vi "Microwave Oven.vi"(0 "Key_Pad":T2 caption="Key Pad", 5 "Stop":bool, 7 "Door_Open":bool caption="Door Open") -> (4 "Display_Panel":string caption="Display Panel", 6 "Recipe":string[][](table), 8 "Oven_Data_Display":T1 caption="Microwave Oven")   [LabVIEW 2023]
doc: "This VI is the Main VI that performs the oven operations."
uses:
  Controls/Key_Pad.ctl
  Controls/Oven_Data_Display.ctl
  Controls/Oven_Data.ctl
  Controls/Timer_Operation_Select.ctl
  Controls/Timer_Data.ctl
  Controls/Queue_Operation_Select.ctl
  <vilib>/Utility/file.llb/Read Delimited Spreadsheet (string).vi
panel:
  out "Error_Out":errorcluster
  in  "Error_In":errorcluster
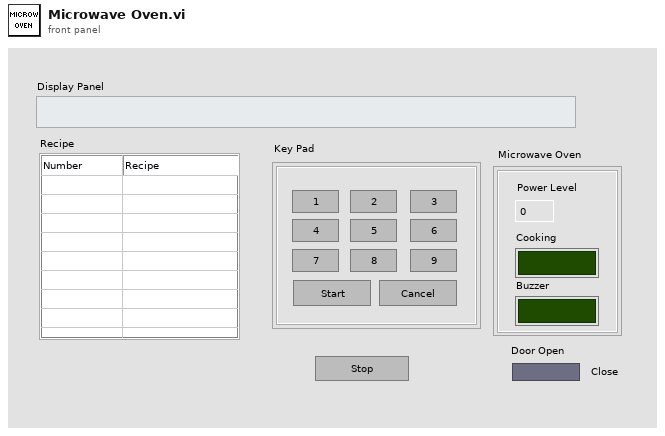
[diagram p1: front panel]
types:
  T1 = typedef "Oven_Data_Display.ctl" = cluster{"Power_Level":i32, "Cooking":bool, "Buzzer":bool}
  T2 = typedef "Key_Pad.ctl" = cluster{"One":bool, "Two":bool, "Three":bool, "Four":bool, "Five":bool, "Six":bool, "Seven":bool, "Eight":bool, "Nine":bool, "Start":bool, "Cancel":bool}
  T3 = typedef "Queue_Operation_Select.ctl" = enum16{"Obtain_Queue", "Enqueue", "Enqueue_at_First", "Enqueue_N", "Dequeue", "Flush_Queue", "Release_Queue"}
  T4 = typedef "Oven_Data.ctl" = cluster{"Recipe_Data":string[][], "Display_Message":string, "Recipe_Code":i32, "Start?":bool, "Cancel?":bool, "TimeOut?":bool, "Door_Open?":bool, "Cooking_Completed?":bool, "Current_Stage":i32, "Timer_Operation_Select":T5, "Oven_Data_Display":T1, "Recipe_Data_Dispaly":string[][], "Total_Stage":i32, "Timer_Data":T6, "Recipe_Selected":string}
  T5 = typedef "Timer_Operation_Select.ctl" = enum16{"Start_Timer", "Pause_Timer", "Stop_Timer", "CheckOut_Timer"}
  T6 = typedef "Timer_Data.ctl" = cluster{"Present_Time":dbl, "Start?":bool, "Time_Before_Pause":dbl, "Time_Required":dbl, "Time":dbl}
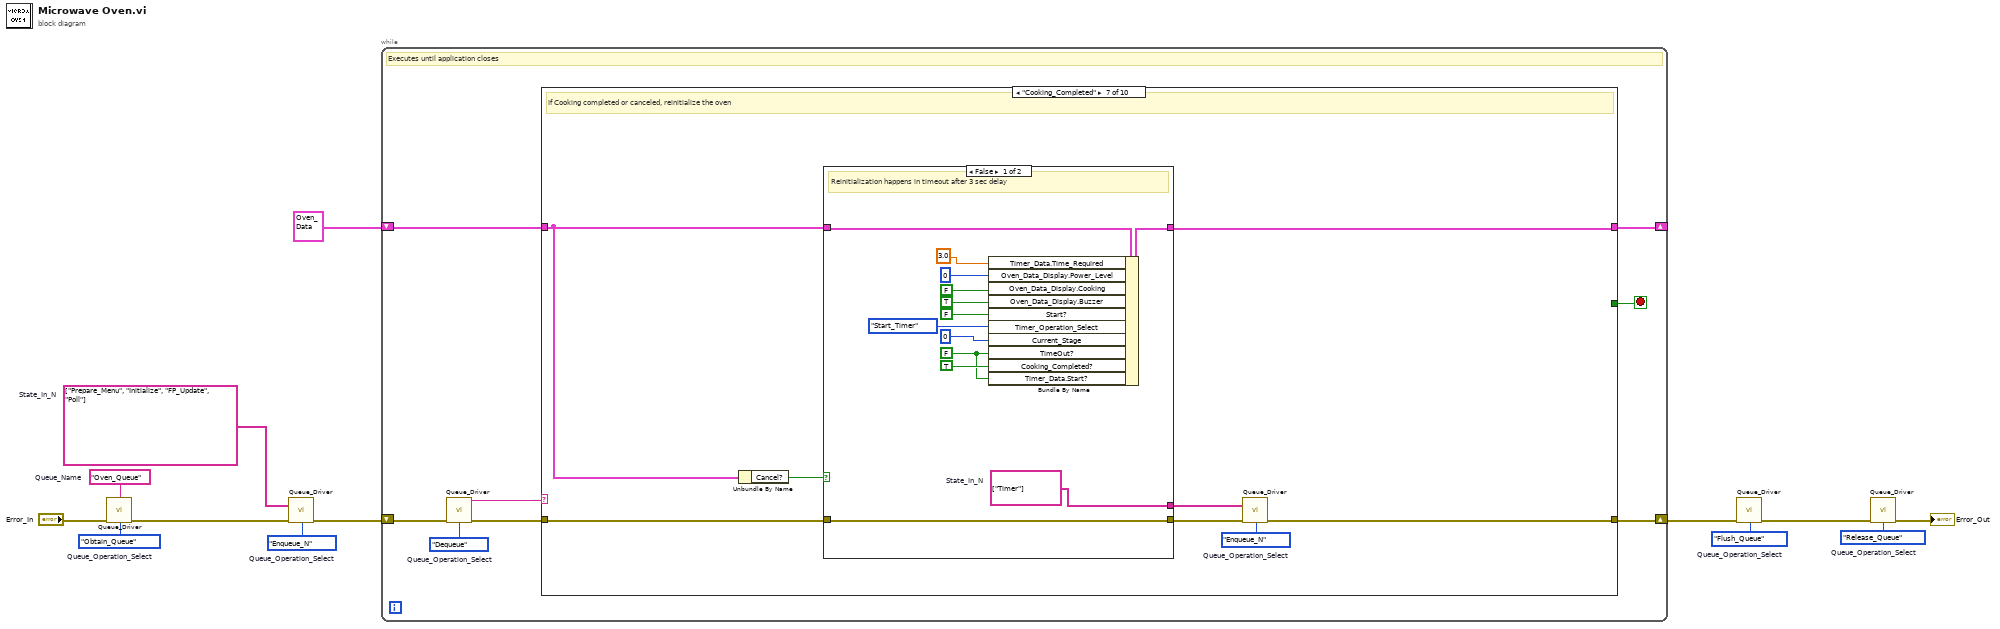
[diagram p0: block diagram]
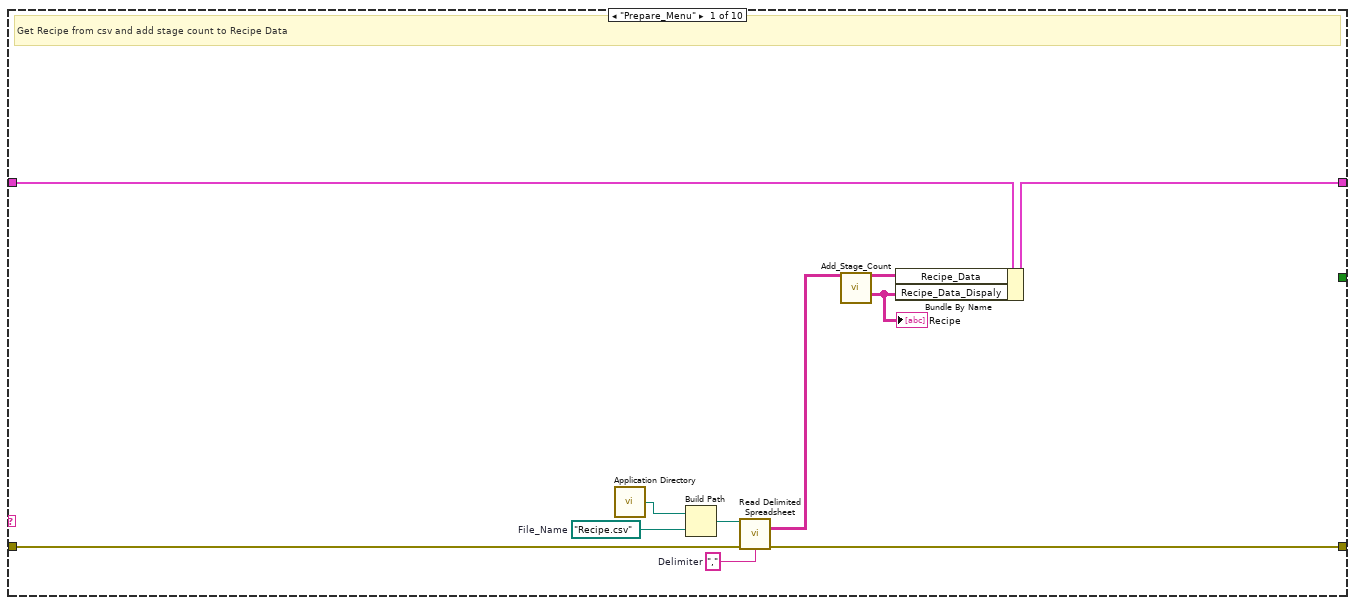
[diagram p2: hidden frame]
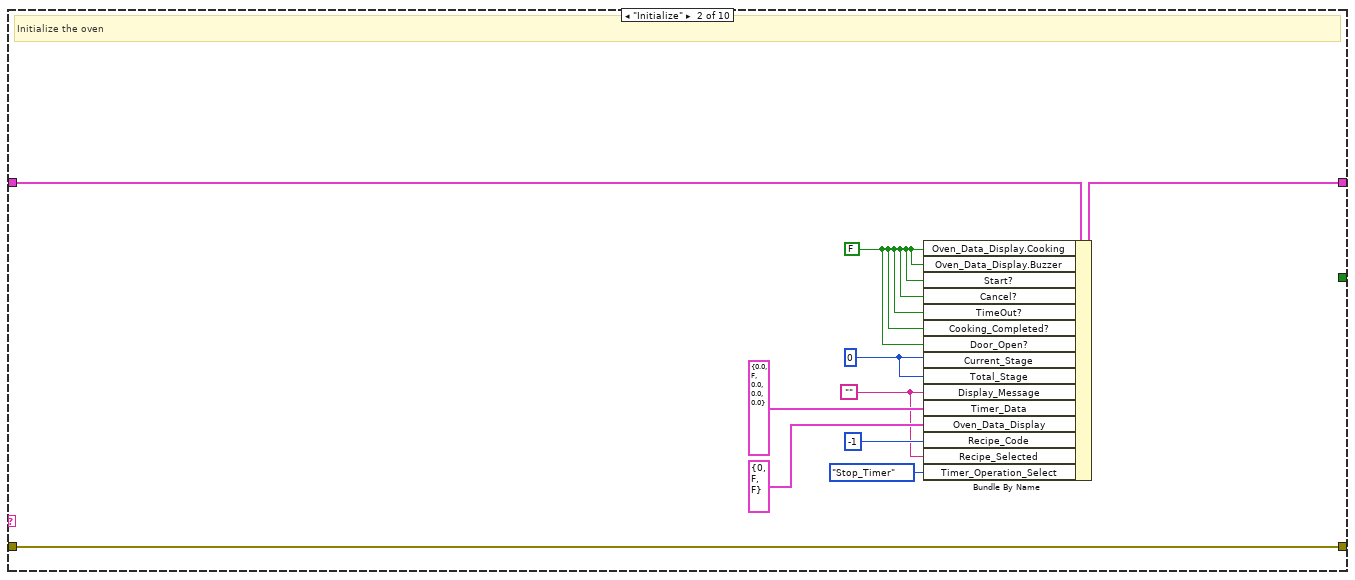
[diagram p3: hidden frame]
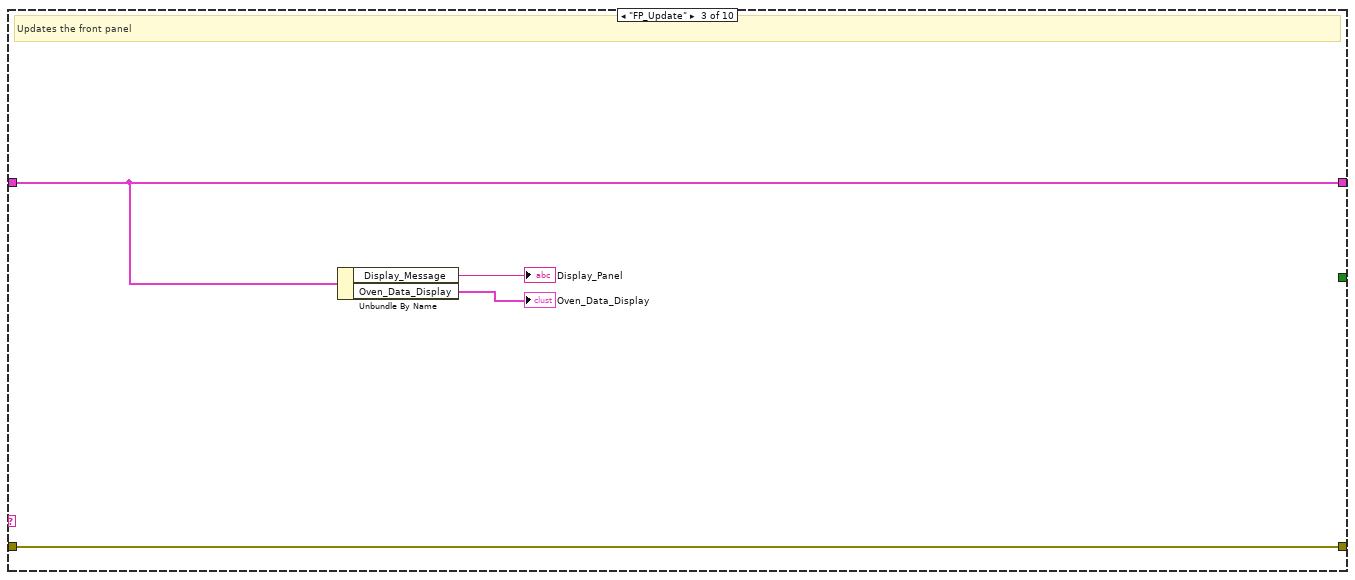
[diagram p4: hidden frame]
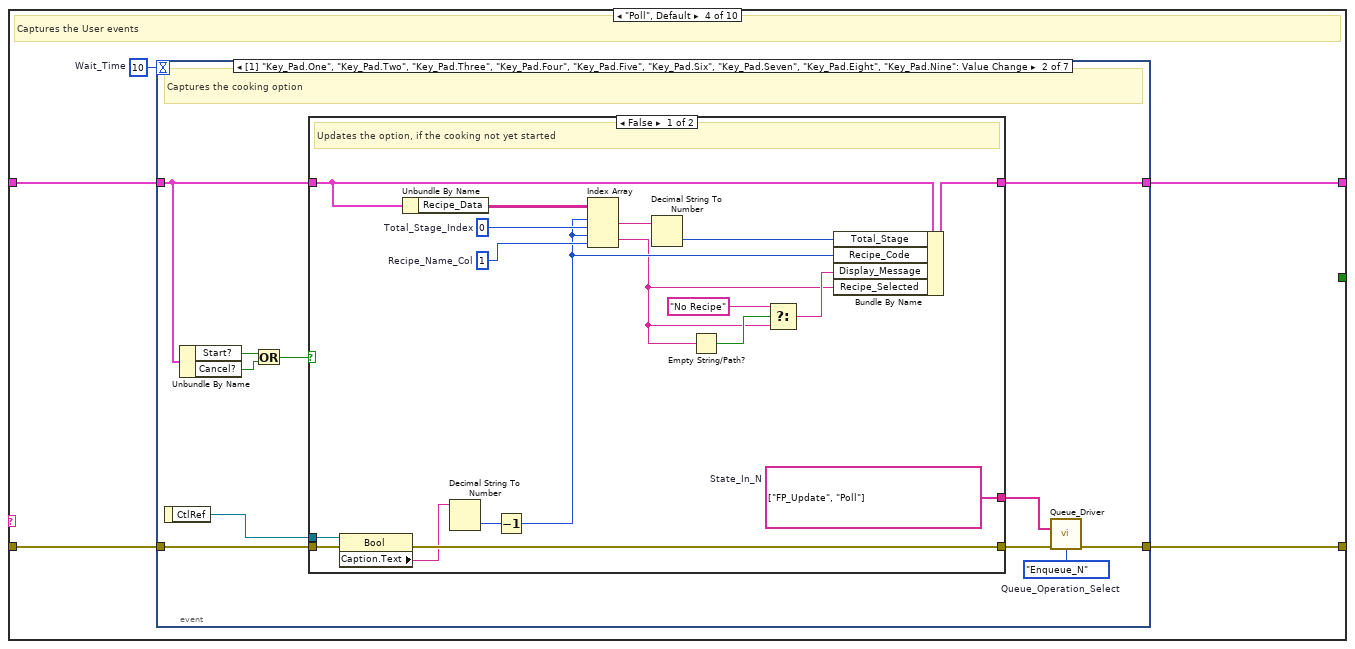
[diagram p5: hidden frame]
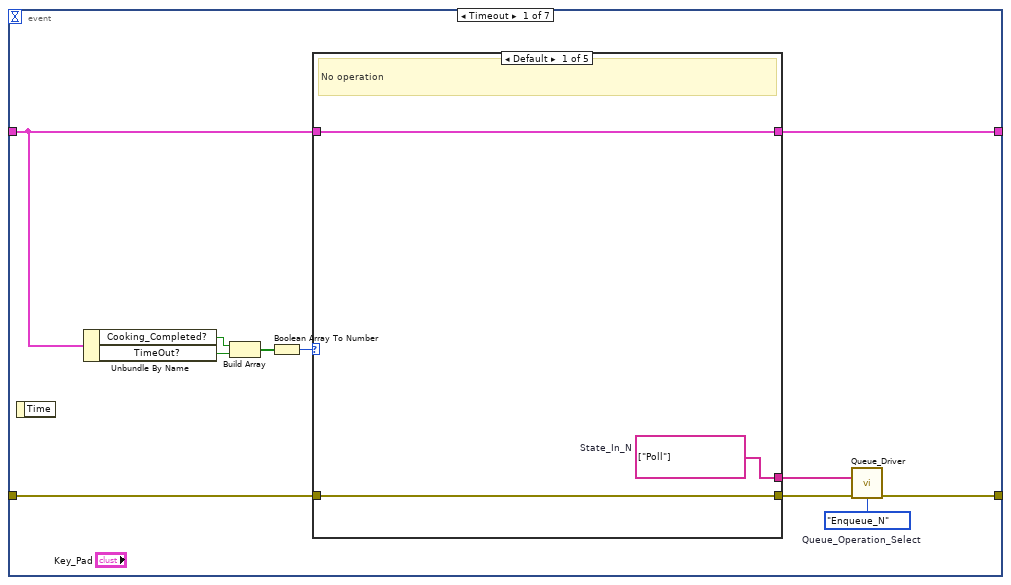
[diagram p6: hidden frame]
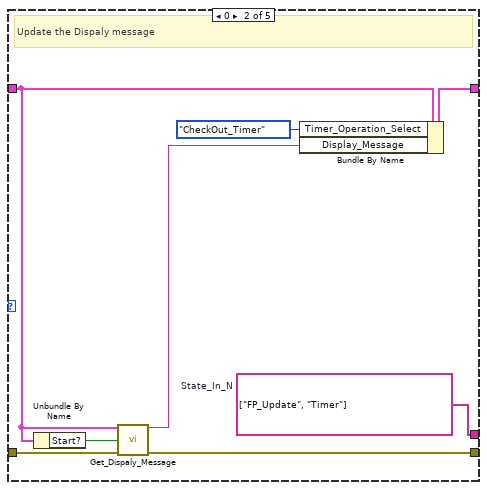
[diagram p7: hidden frame]
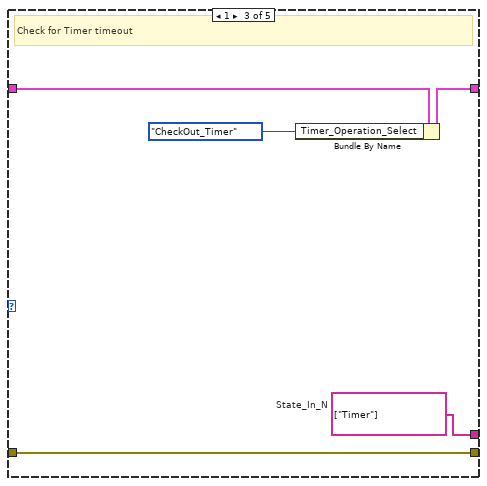
[diagram p8: hidden frame]
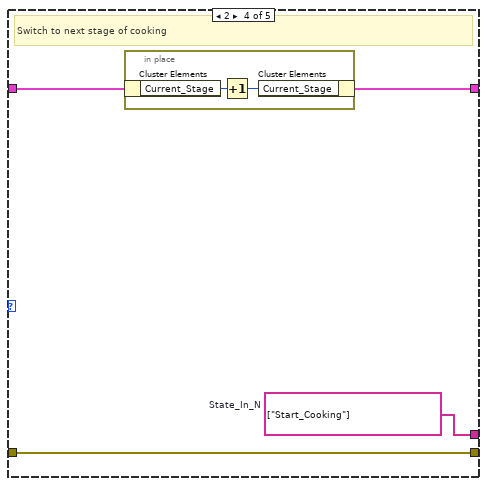
[diagram p9: hidden frame]
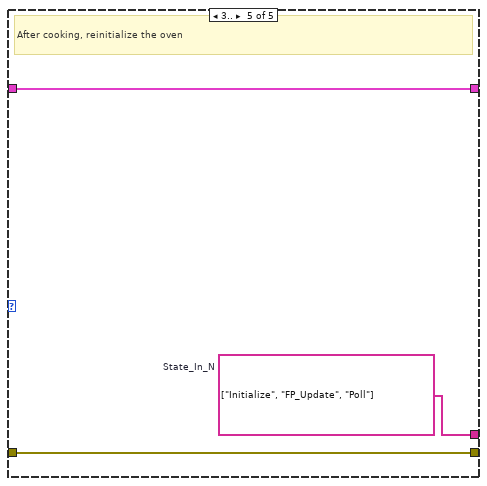
[diagram p10: hidden frame]
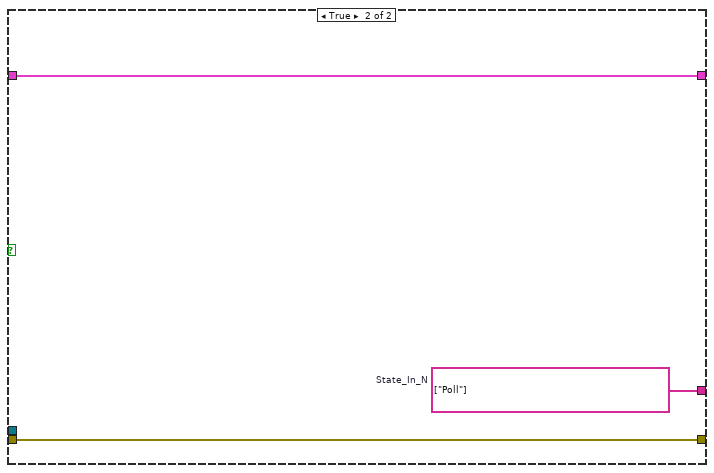
[diagram p11: hidden frame]
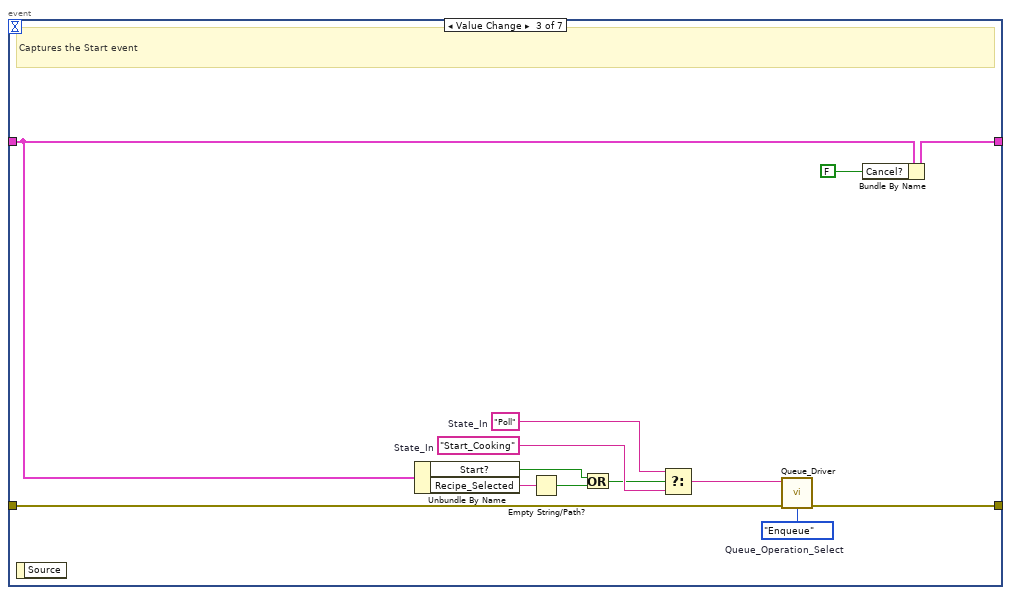
[diagram p12: hidden frame]
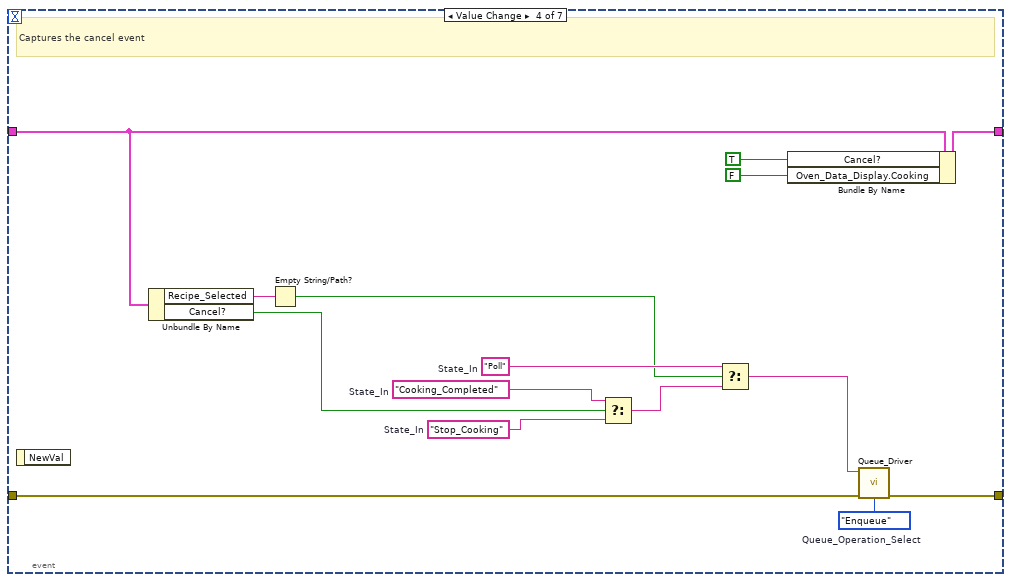
[diagram p13: hidden frame]
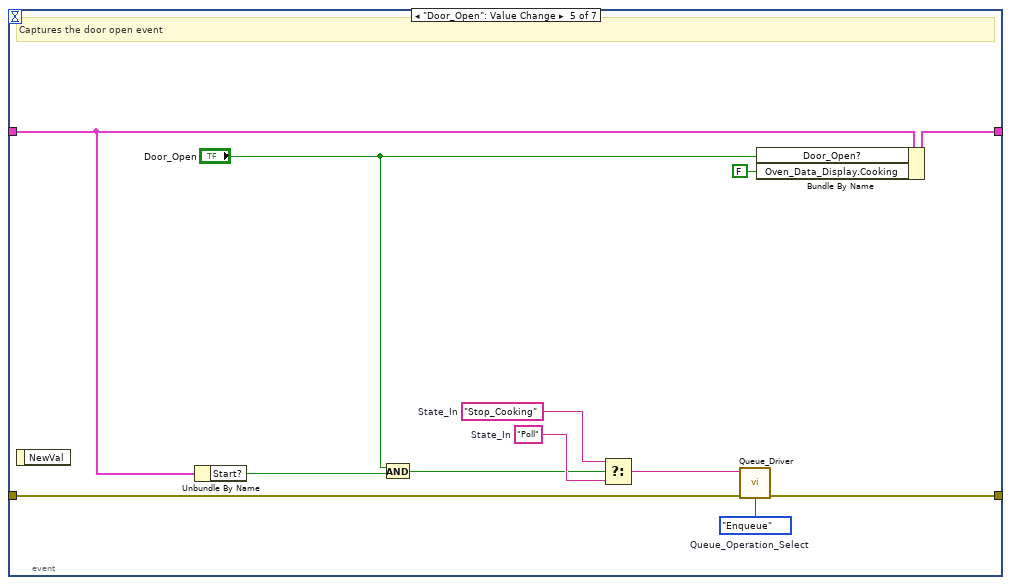
[diagram p14: hidden frame]
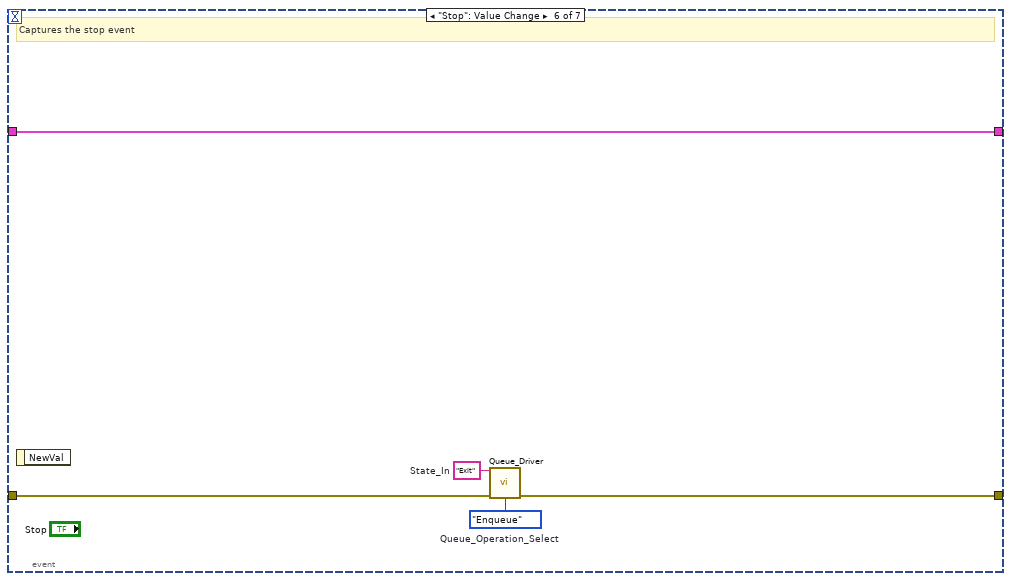
[diagram p15: hidden frame]
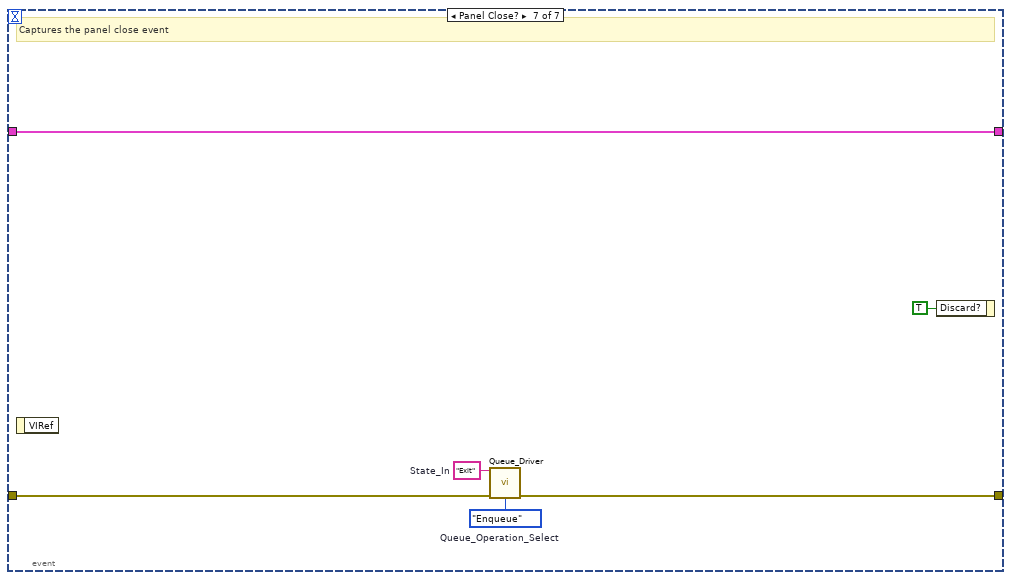
[diagram p16: hidden frame]
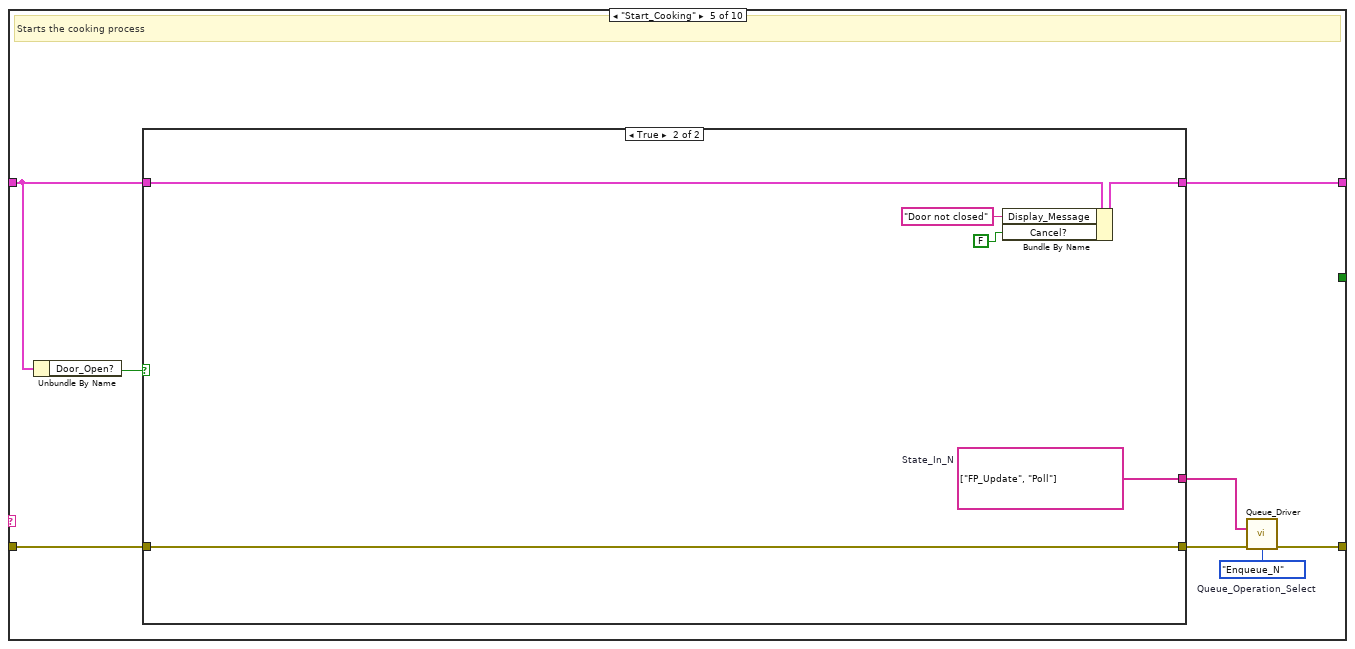
[diagram p17: hidden frame]
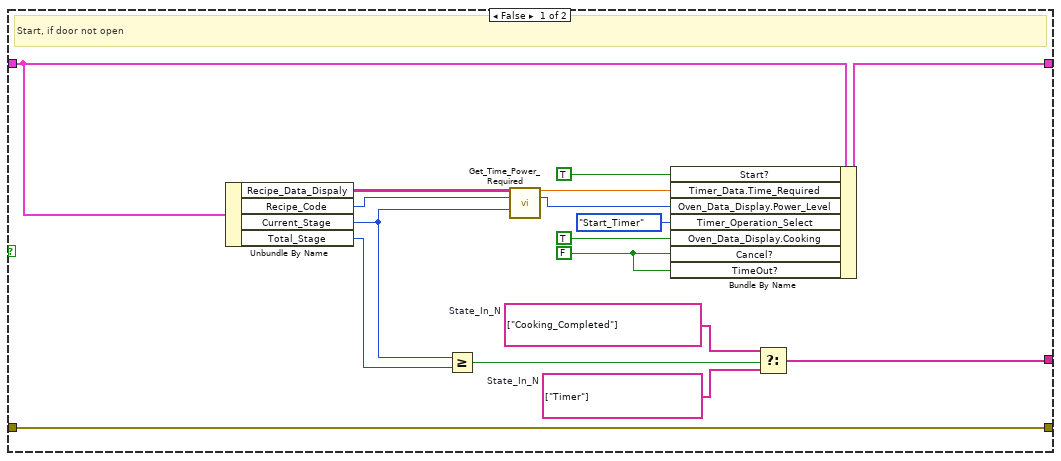
[diagram p18: hidden frame]
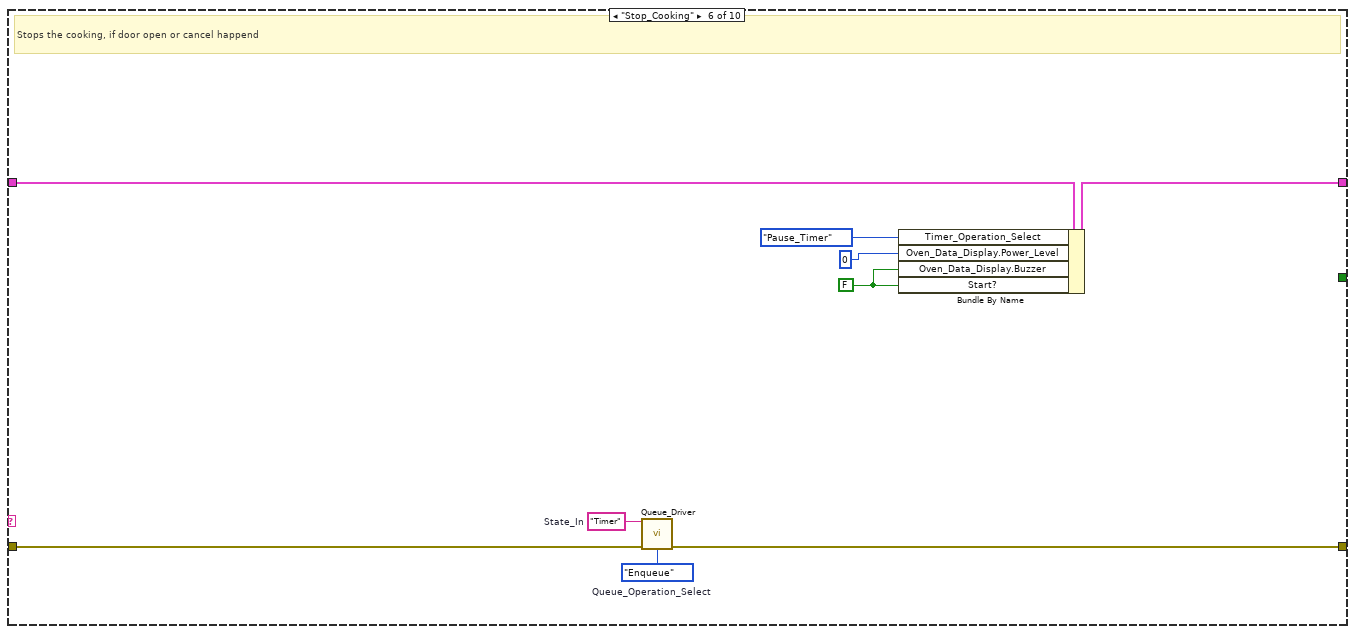
[diagram p19: hidden frame]
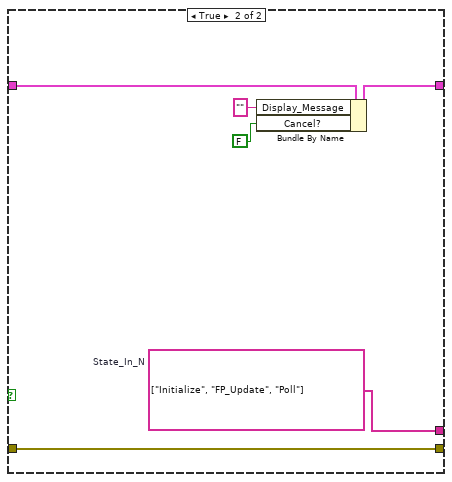
[diagram p20: hidden frame]
diagram:
  w1 = Queue_Operation_Select."Release_Queue"  # Queue_Operation_Select
  w2 = Queue_Operation_Select."Flush_Queue"  # Queue_Operation_Select
  w5 = string[] ["Prepare_Menu", "Initialize", "FP_Update", "Poll"]  # State_In_N
  w6 = Queue_Operation_Select."Enqueue_N"  # Queue_Operation_Select
  w8 = "Oven_Queue"  # Queue_Name
  w9 = Queue_Operation_Select."Obtain_Queue"  # Queue_Operation_Select
  n1 = call "Queue_Driver.vi"("Queue_Name"=w8, "Error_In"="Error_In", "Queue_Operation_Select"=w9) -> ("Error_Out"=w10:errorcluster)  [unwired: 11 in, 1 out]
  n2 = call "Queue_Driver.vi"("State_In_N"=w5, "Error_In"=w10, "Queue_Operation_Select"=w6) -> ("Error_Out"=w7:errorcluster)  [unwired: 11 in, 1 out]
  n3 = while {
    shift-right: [w19] -> _
    shift-left: T4 {"Recipe_Data"=[], "Display_Message"="", "Recipe_Code"=0, "Start?"=FALSE, "Cancel?"=FALSE, "TimeOut?"=FALSE, "Door_Open?"=FALSE, "Cooking_Completed?"=FALSE, "Current_Stage"=0, "Timer_Operation_Select"=enum."CheckOut_Timer", "Oven_Data_Display"={"Power_Level"=0, "Cooking"=FALSE, "Buzzer"=FALSE}, "Recipe_Data_Dispaly"=[], "Total_Stage"=0, "Timer_Data"={"Present_Time"=0.0, "Start?"=FALSE, "Time_Before_Pause"=0.0, "Time_Required"=0.0, "Time"=0.0}, "Recipe_Selected"=""} -> [w18]
    shift-right: [w20] -> w12
    shift-left: w7 -> [w21]
    stop <- w14 stop-if-true
    w16 = Queue_Operation_Select."Dequeue"  # Queue_Operation_Select
    # "Executes until application closes"
    n4 = call "Queue_Driver.vi"("Error_In"=w21, "Queue_Operation_Select"=w16) -> ("State_Out"=w15:string, "Error_Out"=w17:errorcluster)  [unwired: 12 in]
    n5 = case shown="\"Cooking_Completed\"" w15 {
      tunnel: w17 -> [w31 w42 w46 w50 w176 w210 w215 w243 w250 w259]
      tunnel: [w30 w42 w46 w51 w173 w209 w218 w240 w250 w258] -> w20
      tunnel: [w25 w41 w45 w49 w178 w206 w213 w241 w249 w270] -> w19
      tunnel: w18 -> [w32 w40 w45 w48 w175 w202 w212 w244 w249 w270]
      tunnel: [_ _ _ _ _ _ _ _ w245 _] -> w14
      frame "Prepare_Menu" {
        w26 = ","  # Delimiter
        w27 = path "Recipe.csv"  # File_Name
        # "Get Recipe from csv and add stage count to Recipe Data"
        n6 = call <vilib>:"Application Directory.vi"() -> ("Application Directory"=w28:path)
        n7 = Build Path(base path=w28, name or relative path=w27) -> (appended path=w29:path)
        n8 = call-poly <vilib>:"Read Delimited Spreadsheet.vi"("file path (dialog if empty)"=w29, "error in (no error)"=w31, "delimiter (\\t)"=w26) -> ("all rows"=w24:string[][], "error out"=w30:errorcluster)  [unwired: 7 in, 4 out]
        n9 = call "Add_Stage_Count.vi"("Recipe_Data"=w24) -> ("Recipe_Data_with_StageCount"=w23:string[][], "Recipe_Data_Display"=w22:string[][])  [unwired: 13 in]
        "Recipe" <- w22
        n10 = Bundle By Name(cluster=w32, "Recipe_Data"=w23, "Recipe_Data_Dispaly"=w22) -> (w25:T4)
      }
      frame "Initialize" {
        w33 = "" ("Empty String Constant")
        w39 = 0 ("Current_Stage")
        w34 = FALSE ("Start?")
        # "Initialize the oven"
        n11 = Bundle By Name(cluster=w40, "Oven_Data_Display.Cooking"=w34, "Oven_Data_Display.Buzzer"=w34, "Start?"=w34, "Cancel?"=w34, "TimeOut?"=w34, "Cooking_Completed?"=w34, "Door_Open?"=w34, "Current_Stage"=w39, "Total_Stage"=w39, "Display_Message"=w33, "Timer_Data"=T6 {"Present_Time"=0.0, "Start?"=FALSE, "Time_Before_Pause"=0.0, "Time_Required"=0.0, "Time"=0.0}, "Oven_Data_Display"=T1 {"Power_Level"=0, "Cooking"=FALSE, "Buzzer"=FALSE}, "Recipe_Code"=-1, "Recipe_Selected"=w33, "Timer_Operation_Select"=Timer_Operation_Select."Stop_Timer") -> (w41:T4)
      }
      frame "FP_Update" {
        # "Updates the front panel"
        n12 = Unbundle By Name(w45) -> ("Display_Message"=→"Display_Panel":string, "Oven_Data_Display"=→"Oven_Data_Display":T1)
      }
      frame "Poll", Default {
        w47 = 10  # Wait_Time
        # "Captures the User events"
        n13 = event shown="[1] \"Key_Pad.One\", \"Key_Pad.Two\", \"Key_Pad.Three\", \"Key_Pad.Four\", \"Key_Pad.Five\", \"Key_Pad.Six\", \"Key_Pad.Seven\", \"Key_Pad.Eight\", \"Key_Pad.Nine\": Value Change" {
          selector: _ -> [_ _ _ _ _ _ _]
          dyn-events: _ -> [_ _ _ _ _ _ _]
          timeout: w47 -> [_ _ _ _ _ _ _]
          tunnel: [w62 w94 w131 w147 w158 w162 w167] -> w51
          tunnel: w50 -> [w59 w98 w132 w141 w159 w164 w170]
          tunnel: [w54 w95 w130 w145 w156 w163 w169] -> w49
          tunnel: w48 -> [w53 w91 w125 w146 w151 w163 w169]
          event Timeout {
            w61 = Queue_Operation_Select."Enqueue_N"  # Queue_Operation_Select
            n14 = event-data() -> ()  [unwired: 1 in, 1 out]
            n15 = Unbundle By Name(w53) -> ("Cooking_Completed?"=w52:bool, "TimeOut?"=w57:bool)
            n16 = Build Array(w52, w57) -> (w56:bool[])
            n17 = Boolean Array To Number(Boolean array=w56) -> (number=w55:u32)
            n18 = case shown="Default" w55 {
              tunnel: [w64 w68 w77 w82 w87] -> w60
              tunnel: w59 -> [w64 w69 w77 w82 w87]
              tunnel: [w63 w73 w76 w81 w86] -> w58
              tunnel: [w65 w71 w75 w80 w85] -> w54
              tunnel: w53 -> [w65 w67 w78 w79 w85]
              frame Default {
                w63 = string[] ["Poll"]  # State_In_N
                # "No operation"
              }
              frame 0 {
                w73 = string[] ["FP_Update", "Timer"]  # State_In_N
                # "Update the Dispaly message"
                n19 = Unbundle By Name(w67) -> ("Start?"=w66:bool)
                n20 = call "Get_Dispaly_Message.vi"("Oven_Data"=w67, "Start?"=w66, "Error_In"=w69) -> ("Message_Display"=w70:string, "Error_Out"=w68:errorcluster)  [unwired: 11 in]
                n21 = Bundle By Name(cluster=w67, "Timer_Operation_Select"=Timer_Operation_Select."CheckOut_Timer", "Display_Message"=w70) -> (w71:T4)
              }
              frame 1 {
                w76 = string[] ["Timer"]  # State_In_N
                # "Check for Timer timeout"
                n22 = Bundle By Name(cluster=w78, "Timer_Operation_Select"=Timer_Operation_Select."CheckOut_Timer") -> (w75:T4)
              }
              frame 2 {
                w81 = string[] ["Start_Cooking"]  # State_In_N
                # "Switch to next stage of cooking"
                n23 = in-place "In Place Element Structure" {
                  n24 = in-place-cluster #1(w79) -> ("Current_Stage"=w84:i32)
                  n25 = Increment(x=w84) -> (x+1=w83:i32)
                  n26 = in-place-cluster #1("Current_Stage"=w83) -> (w80:T4)
                }
              }
              frame 3.. {
                w86 = string[] ["Initialize", "FP_Update", "Poll"]  # State_In_N
                # "After cooking, reinitialize the oven"
              }
            }
            n27 = call "Queue_Driver.vi"("State_In_N"=w58, "Error_In"=w60, "Queue_Operation_Select"=w61) -> ("Error_Out"=w62:errorcluster)  [unwired: 11 in, 1 out]
          }
          event Value Change {
            w93 = Queue_Operation_Select."Enqueue_N"  # Queue_Operation_Select
            # "Captures the cooking option"
            n28 = event-data() -> ("CtlRef"=w96:refnum<vi>)  [unwired: 1 in]
            n29 = Unbundle By Name(w91) -> ("Start?"=w90:bool, "Cancel?"=w88:bool)
            n30 = Or(x=w90, y=w88) -> (x .or. y?=w89:bool)
            n31 = case shown="False" w89 {
              tunnel: w98 -> [w116 w118]
              tunnel: [w115 w118] -> w97
              tunnel: w96 -> [w114 _]
              tunnel: w91 -> [w112 w119]
              tunnel: [w110 w119] -> w95
              tunnel: [w109 w117] -> w92
              frame False {
                w106 = 0  # Total_Stage_Index
                w109 = string[] ["FP_Update", "Poll"]  # State_In_N
                w108 = 1  # Recipe_Name_Col
                # "Updates the option, if the cooking not yet started"
                n32 = property on="Property Node" class="Bool"(reference=w114, error in=w116) -> (error out=w115:errorcluster, "Caption.Text"=w113:string)  [unwired: 1 out]
                n33 = Unbundle By Name(w112) -> ("Recipe_Data"=w111:string[][])
                n34 = Decimal String To Number(string=w113) -> (number=w107:i32)  [unwired: 2 in, 1 out]
                n35 = Decrement(x=w107) -> (x-1=w103:i32)
                n36 = Index Array(array=w111, index (row) #1=w103, index (col) #1=w106, index (row) #2=w103, index (col) #2=w108) -> (element #1=w105:string, element #2=w99:string)
                n37 = Decimal String To Number(string=w105) -> (number=w104:i32)  [unwired: 2 in, 1 out]
                n38 = Empty String/Path?(string/path=w99) -> (empty?=w102:bool)
                n39 = Select(t="No Recipe", s=w102, f=w99) -> (s? t:f=w100:string)
                n40 = Bundle By Name(cluster=w112, "Total_Stage"=w104, "Recipe_Code"=w103, "Display_Message"=w100, "Recipe_Selected"=w99) -> (w110:T4)
              }
              frame True {
                w117 = string[] ["Poll"]  # State_In_N
              }
            }
            n41 = call "Queue_Driver.vi"("State_In_N"=w92, "Error_In"=w97, "Queue_Operation_Select"=w93) -> ("Error_Out"=w94:errorcluster)  [unwired: 11 in, 1 out]
          }
          event Value Change {
            w127 = "Poll"  # State_In
            w128 = "Start_Cooking"  # State_In
            w129 = Queue_Operation_Select."Enqueue"  # Queue_Operation_Select
            # "Captures the Start event"
            n42 = event-data() -> ()  [unwired: 1 in, 1 out]
            n43 = Unbundle By Name(w125) -> ("Start?"=w124:bool, "Recipe_Selected"=w122:string)
            n44 = Empty String/Path?(string/path=w122) -> (empty?=w121:bool)
            n45 = Or(x=w124, y=w121) -> (x .or. y?=w123:bool)
            n46 = Select(t=w127, s=w123, f=w128) -> (s? t:f=w120:string)
            n47 = call "Queue_Driver.vi"("State_In"=w120, "Error_In"=w132, "Queue_Operation_Select"=w129) -> ("Error_Out"=w131:errorcluster)  [unwired: 11 in, 1 out]
            n48 = Bundle By Name(cluster=w125, "Cancel?"=FALSE) -> (w130:T4)
          }
          event Value Change {
            w137 = "Poll"  # State_In
            w143 = "Cooking_Completed"  # State_In
            w139 = "Stop_Cooking"  # State_In
            w142 = Queue_Operation_Select."Enqueue"  # Queue_Operation_Select
            # "Captures the cancel event"
            n49 = event-data() -> ()  [unwired: 1 in, 1 out]
            n50 = Unbundle By Name(w146) -> ("Recipe_Selected"=w134:string, "Cancel?"=w133:bool)
            n51 = Empty String/Path?(string/path=w134) -> (empty?=w136:bool)
            n52 = Select(t=w143, s=w133, f=w139) -> (s? t:f=w138:string)
            n53 = Select(t=w137, s=w136, f=w138) -> (s? t:f=w135:string)
            n54 = Bundle By Name(cluster=w146, "Cancel?"=TRUE, "Oven_Data_Display.Cooking"=FALSE) -> (w145:T4)
            n55 = call "Queue_Driver.vi"("State_In"=w135, "Error_In"=w141, "Queue_Operation_Select"=w142) -> ("Error_Out"=w147:errorcluster)  [unwired: 11 in, 1 out]
          }
          event "Door_Open": Value Change {
            w152 = "Poll"  # State_In
            w154 = "Stop_Cooking"  # State_In
            w157 = Queue_Operation_Select."Enqueue"  # Queue_Operation_Select
            # "Captures the door open event"
            n56 = event-data() -> ()  [unwired: 1 in, 1 out]
            n57 = Unbundle By Name(w151) -> ("Start?"=w150:bool)
            n58 = And(x="Door_Open", y=w150) -> (x .and. y?=w149:bool)
            n59 = Select(t=w154, s=w149, f=w152) -> (s? t:f=w153:string)
            n60 = call "Queue_Driver.vi"("State_In"=w153, "Error_In"=w159, "Queue_Operation_Select"=w157) -> ("Error_Out"=w158:errorcluster)  [unwired: 11 in, 1 out]
            n61 = Bundle By Name(cluster=w151, "Door_Open?"="Door_Open", "Oven_Data_Display.Cooking"=FALSE) -> (w156:T4)
          }
          event "Stop": Value Change {
            w160 = "Exit"  # State_In
            w161 = Queue_Operation_Select."Enqueue"  # Queue_Operation_Select
            # "Captures the stop event"
            n62 = event-data() -> ()  [unwired: 1 in, 1 out]
            n63 = call "Queue_Driver.vi"("State_In"=w160, "Error_In"=w164, "Queue_Operation_Select"=w161) -> ("Error_Out"=w162:errorcluster)  [unwired: 11 in, 1 out]
          }
          event Panel Close? {
            w165 = "Exit"  # State_In
            w166 = Queue_Operation_Select."Enqueue"  # Queue_Operation_Select
            # "Captures the panel close event"
            n64 = event-data() -> ()  [unwired: 1 in, 1 out]
            n65 = call "Queue_Driver.vi"("State_In"=w165, "Error_In"=w170, "Queue_Operation_Select"=w166) -> ("Error_Out"=w167:errorcluster)  [unwired: 11 in, 1 out]
            n66 = event-data ("Event Filter Node")("Discard?"=TRUE) -> ()  [unwired: 1 in, 1 out]
          }
        }
      }
      frame "Start_Cooking" {
        w172 = Queue_Operation_Select."Enqueue_N"  # Queue_Operation_Select
        # "Starts the cooking process"
        n67 = Unbundle By Name(w175) -> ("Door_Open?"=w174:bool)
        n68 = case shown="True" w174 {
          tunnel: w175 -> [w195 w201]
          tunnel: [w193 w200] -> w178
          tunnel: [w189 w197] -> w177
          tunnel: w176 -> [w189 w197]
          tunnel: [w182 w196] -> w171
          frame False {
            w179 = string[] ["Timer"]  # State_In_N
            w180 = string[] ["Cooking_Completed"]  # State_In_N
            w184 = FALSE ("Cancel?")
            # "Start, if door not open"
            n69 = Unbundle By Name(w195) -> ("Recipe_Data_Dispaly"=w194:string[][], "Recipe_Code"=w185:i32, "Current_Stage"=w186:i32, "Total_Stage"=w188:i32)
            n70 = Greater Or Equal?(x=w186, y=w188) -> (x >= y?=w181:bool)
            n71 = call "Get_Time_Power_Required.vi"("Recipe_Data_Dispaly"=w194, "Recipe_Code"=w185, "Current_Stage"=w186) -> ("Time_Required"=w183:dbl, "Power_Required"=w192:i32)  [unwired: 11 in]
            n72 = Bundle By Name(cluster=w195, "Start?"=TRUE, "Timer_Data.Time_Required"=w183, "Oven_Data_Display.Power_Level"=w192, "Timer_Operation_Select"=Timer_Operation_Select."Start_Timer", "Oven_Data_Display.Cooking"=TRUE, "Cancel?"=w184, "TimeOut?"=w184) -> (w193:T4)
            n73 = Select(t=w180, s=w181, f=w179) -> (s? t:f=w182:string[])
          }
          frame True {
            w196 = string[] ["FP_Update", "Poll"]  # State_In_N
            n74 = Bundle By Name(cluster=w201, "Display_Message"="Door not closed", "Cancel?"=FALSE) -> (w200:T4)
          }
        }
        n75 = call "Queue_Driver.vi"("State_In_N"=w171, "Error_In"=w177, "Queue_Operation_Select"=w172) -> ("Error_Out"=w173:errorcluster)  [unwired: 11 in, 1 out]
      }
      frame "Stop_Cooking" {
        w203 = FALSE ("Oven_Data_Display.Buzzer")
        w207 = "Timer"  # State_In
        w208 = Queue_Operation_Select."Enqueue"  # Queue_Operation_Select
        # "Stops the cooking, if door open or cancel happend"
        n76 = call "Queue_Driver.vi"("State_In"=w207, "Error_In"=w210, "Queue_Operation_Select"=w208) -> ("Error_Out"=w209:errorcluster)  [unwired: 11 in, 1 out]
        n77 = Bundle By Name(cluster=w202, "Timer_Operation_Select"=Timer_Operation_Select."Pause_Timer", "Oven_Data_Display.Power_Level"=0, "Oven_Data_Display.Buzzer"=w203, "Start?"=w203) -> (w206:T4)
      }
      frame "Cooking_Completed" {
        w217 = Queue_Operation_Select."Enqueue_N"  # Queue_Operation_Select
        # "If Cooking completed or canceled, reinitialize the oven"
        n78 = Unbundle By Name(w212) -> ("Cancel?"=w211:bool)
        n79 = case shown="False" w211 {
          tunnel: [w230 w237] -> w216
          tunnel: w215 -> [w231 w236]
          tunnel: [w231 w236] -> w214
          tunnel: [w229 w234] -> w213
          tunnel: w212 -> [w224 w235]
          frame False {
            w219 = FALSE ("TimeOut?")
            w230 = string[] ["Timer"]  # State_In_N
            # "Reinitialization happens in timeout after 3 sec delay"
            n80 = Bundle By Name(cluster=w224, "Timer_Data.Time_Required"=3.0 ("Time_Required"), "Oven_Data_Display.Power_Level"=0, "Oven_Data_Display.Cooking"=FALSE, "Oven_Data_Display.Buzzer"=TRUE, "Start?"=FALSE, "Timer_Operation_Select"=Timer_Operation_Select."Start_Timer", "Current_Stage"=0, "TimeOut?"=w219, "Cooking_Completed?"=TRUE, "Timer_Data.Start?"=w219) -> (w229:T4)
          }
          frame True {
            w237 = string[] ["Initialize", "FP_Update", "Poll"]  # State_In_N
            n81 = Bundle By Name(cluster=w235, "Display_Message"="", "Cancel?"=FALSE) -> (w234:T4)
          }
        }
        n82 = call "Queue_Driver.vi"("State_In_N"=w216, "Error_In"=w214, "Queue_Operation_Select"=w217) -> ("Error_Out"=w218:errorcluster)  [unwired: 11 in, 1 out]
      }
      frame "Timer" {
        w238 = string[] ["FP_Update", "Poll"]  # State_In_N
        w239 = Queue_Operation_Select."Enqueue_N"  # Queue_Operation_Select
        # "Timer used to maintain the delay in cooking"
        n83 = call "Timer.vi"("Oven_Data_In"=w244, "Error_In"=w243) -> ("Oven_Data_Out"=w241:T4, "Error_Out"=w242:errorcluster)  [unwired: 12 in]
        n84 = call "Queue_Driver.vi"("State_In_N"=w238, "Error_In"=w242, "Queue_Operation_Select"=w239) -> ("Error_Out"=w240:errorcluster)  [unwired: 11 in, 1 out]
      }
      frame "Exit" {
        w248 = "No"  # Back
        w247 = "Yes"  # Stop_Execution
        # "Exit the Application"
        n85 = disable-structure "Conditional Disable Structure" shown="Default" {
          disable-tunnel: [w251 "Do you want to Exit" ("Message")] -> w246
          frame condition #0 (active) {
            w251 = "Do you want to stop the execution"  # Message
            # "Developer mode"
          }
          frame condition #1 {
            # "Real time engine mode"
          }
        }
        n86 = Two Button Dialog(message=w246, 1:w248, 2:w247) -> (T button?=w245:bool)
      }
      frame "Error_State" {
        w254 = "Poll"  # State_In
        w256 = "Exit"  # State_In
        w257 = Queue_Operation_Select."Enqueue"  # Queue_Operation_Select
        w265 = "%d%s%s"  # Format_String
        w266 = "Application Error"  # Initial_String
        w267 = "Stop"  # T_Button
        w268 = "Continue"  # F_Button
        # "Handles error"
        n87 = call <vilib>:"Clear Errors.vi"("error in (no error)"=w259) -> ("error out"=w263:errorcluster)  [unwired: 5 in, 1 out]
        n88 = Unbundle By Name(w259) -> ("code"=w262:i32, "source"=w261:string)
        n89 = Format Into String(format string=w265, initial string=w266, error in=w263, w262, "\n" ("Line Feed Constant"), w261) -> (resulting string=w269:string, error out=w260:errorcluster)
        n90 = Two Button Dialog(message=w269, 1:w268, 2:w267) -> (T button?=w253:bool)
        n91 = Select(t=w256, s=w253, f=w254) -> (s? t:f=w255:string)
        n92 = call "Queue_Driver.vi"("State_In"=w255, "Error_In"=w260, "Queue_Operation_Select"=w257) -> ("Error_Out"=w258:errorcluster)  [unwired: 11 in, 1 out]
      }
    }
  }
  n93 = call "Queue_Driver.vi"("Error_In"=w12, "Queue_Operation_Select"=w2) -> ("Error_Out"=w4:errorcluster)  [unwired: 12 in, 1 out]
  n94 = call "Queue_Driver.vi"("Error_In"=w4, "Queue_Operation_Select"=w1) -> ("Error_Out"=→"Error_Out":errorcluster)  [unwired: 12 in, 1 out]
